vi "VHT Subcarrier Mapper.vi"(9 "bandwidth":enum16{"20MHz", "40MHz", "80MHz"}(ring), 10 "frequency offset index":fxp<+/-,9,9>) -> (1 "subcarrier valid":bool, 2 "pilot subcarrier":bool)   [LabVIEW 2020]
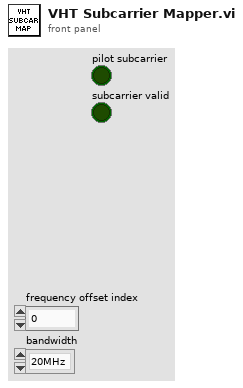
[diagram p1: front panel]
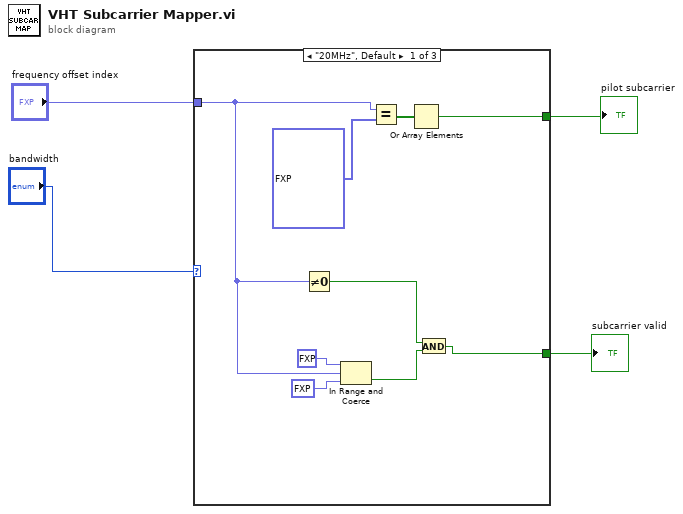
[diagram p0: block diagram]
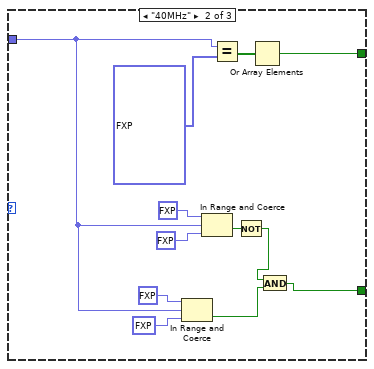
[diagram p2: hidden frame]
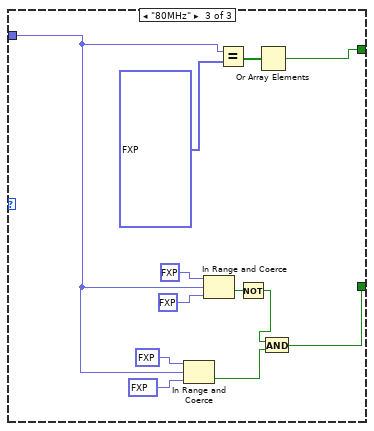
[diagram p3: hidden frame]
diagram:
  n1 = case shown="\"20MHz\", Default" "bandwidth" {
    tunnel: "frequency offset index" -> [w8 w16 w26]
    tunnel: [w11 w20 w28] -> w2
    tunnel: [w5 w19 w27] -> w1
    frame "20MHz", Default {
      n2 = Not Equal To 0?(x=w8) -> (x != 0?=w6:bool)
      n3 = In Range and Coerce(upper limit=fxp<+/-,9,9> 29.0, x=w8, lower limit=fxp<+/-,9,9> -28.0) -> (In Range?=w7:bool)  [unwired: 1 out]
      n4 = Equal?(x=w8, y=fxp<+/-,9,9>[] [-21.0, -7.0, 7.0, 21.0] ("frequency offset index")) -> (x = y?=w12:bool[])
      n5 = Or Array Elements(Boolean array=w12) -> (logical OR=w11:bool)
      n6 = And(x=w6, y=w7) -> (x .and. y?=w5:bool)
    }
    frame "40MHz" {
      n7 = In Range and Coerce(upper limit=fxp<+/-,9,9> 29.0, x=w16, lower limit=fxp<+/-,9,9> -28.0) -> (In Range?=w21:bool)  [unwired: 1 out]
      n8 = In Range and Coerce(upper limit=fxp<+/-,9,9> 2.0, x=w16, lower limit=fxp<+/-,9,9> -1.0) -> (In Range?=w15:bool)  [unwired: 1 out]
      n9 = Equal?(x=w16, y=fxp<+/-,9,9>[] [-53.0, -25.0, -11.0, 11.0, 25.0, 53.0] ("frequency offset index")) -> (x = y?=w24:bool[])
      n10 = Not(x=w15) -> (.not. x?=w14:bool)
      n11 = Or Array Elements(Boolean array=w24) -> (logical OR=w20:bool)
      n12 = And(x=w14, y=w21) -> (x .and. y?=w19:bool)
    }
    frame "80MHz" {
      n13 = In Range and Coerce(upper limit=fxp<+/-,9,9> 123.0, x=w26, lower limit=fxp<+/-,9,9> -122.0) -> (In Range?=w33:bool)  [unwired: 1 out]
      n14 = In Range and Coerce(upper limit=fxp<+/-,9,9> 2.0, x=w26, lower limit=fxp<+/-,9,9> -1.0) -> (In Range?=w30:bool)  [unwired: 1 out]
      n15 = Equal?(x=w26, y=fxp<+/-,9,9>[] [-103.0, -75.0, -39.0, -11.0, 11.0, 39.0, 75.0, 103.0] ("frequency offset index")) -> (x = y?=w36:bool[])
      n16 = Not(x=w30) -> (.not. x?=w29:bool)
      n17 = Or Array Elements(Boolean array=w36) -> (logical OR=w28:bool)
      n18 = And(x=w29, y=w33) -> (x .and. y?=w27:bool)
    }
  }
  "pilot subcarrier" <- w2
  "subcarrier valid" <- w1
